vi "그림 6-3-6 아스키 파일 읽기.vi"() -> ()   [LabVIEW 2010]
panel:
  out "웨이브폼 차트":dbl[][](graph)
  out "배열":dbl[][](array[numeric])
  out "텍스트":string
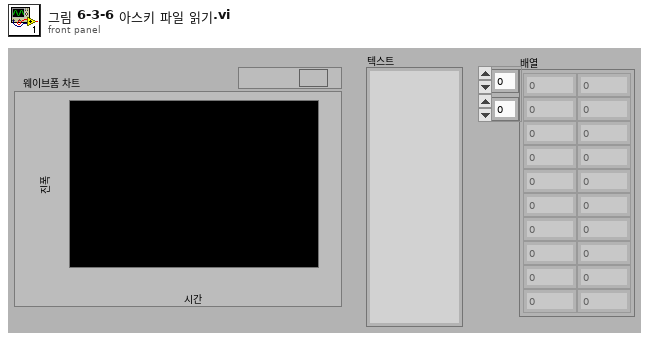
[diagram p1: front panel]
types:
  T1 = enum16{"open", "replace", "create", "open or create", "replace or create", "replace or create with confirmation"}
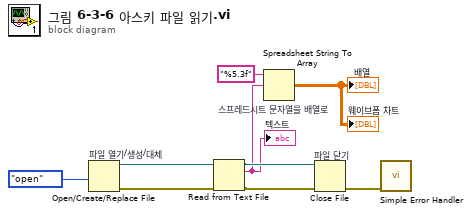
[diagram p0: block diagram]
diagram:
  n1 = Open/Create/Replace File "파일 열기/생성/대체"(operation (0:open)=T1."open" ("동작(0:open)")) -> (refnum out=w7:refnum<file>, error out=w6:errorcluster)  [unwired: 5 in, 1 out]
  n2 = Read from Text File(file (use dialog)=w7, error in=w6) -> (refnum out=w5:refnum<file>, text=w3:string, error out=w4:errorcluster)  [unwired: 2 in, 1 out]
  "텍스트" <- w3
  n3 = Spreadsheet String To Array "스프레드시트 문자열을 배열로"(format string="%5.3f" ("포맷 문자열"), spreadsheet string=w3) -> (array=→"배열" →"웨이브폼 차트":dbl[][])  [unwired: 2 in]
  n4 = Close File "파일 닫기"(refnum=w5, error in=w4) -> (error out=w9:errorcluster)  [unwired: 1 out]
  n5 = call <vilib>:"Simple Error Handler.vi"("error in (no error)"=w9) -> ()  [unwired: 4 in, 5 out]
